vi "Example_scatter.vi"() -> ()   [LabVIEW 8.6]
uses:
  Controls/lxw_chart_marker_type.ctl
  Controls/lxw_chart_legend_position.ctl
  Controls/lxw_chart_axis_type.ctl
  Controls/lxw_chart_type.ctl
panel:
  out "function return 2":string
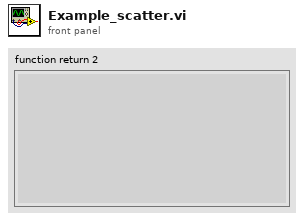
[diagram p1: front panel]
types:
  T1 = enum32{"invalid app kind", "Development System", "Run Time System", "Student Edition", "Embedded LabVIEW", "Evaluation", "Custom"}
  T2 = cluster{"color":u32, "none":u8, "@dummy control@":i8, "@dummy control@":i8, "@dummy control@":i8, "width":sgl, "dash_type":u8, "transparency":u8}
  T3 = cluster{"color":u32, "none":u8, "transparency":u8}
  T4 = typedef "lxw_chart_type.ctl" = u8
  T5 = typedef "lxw_chart_axis_type.ctl" = u8
  T6 = typedef "lxw_chart_legend_position.ctl" = u8
  T7 = typedef "lxw_chart_marker_type.ctl" = u8
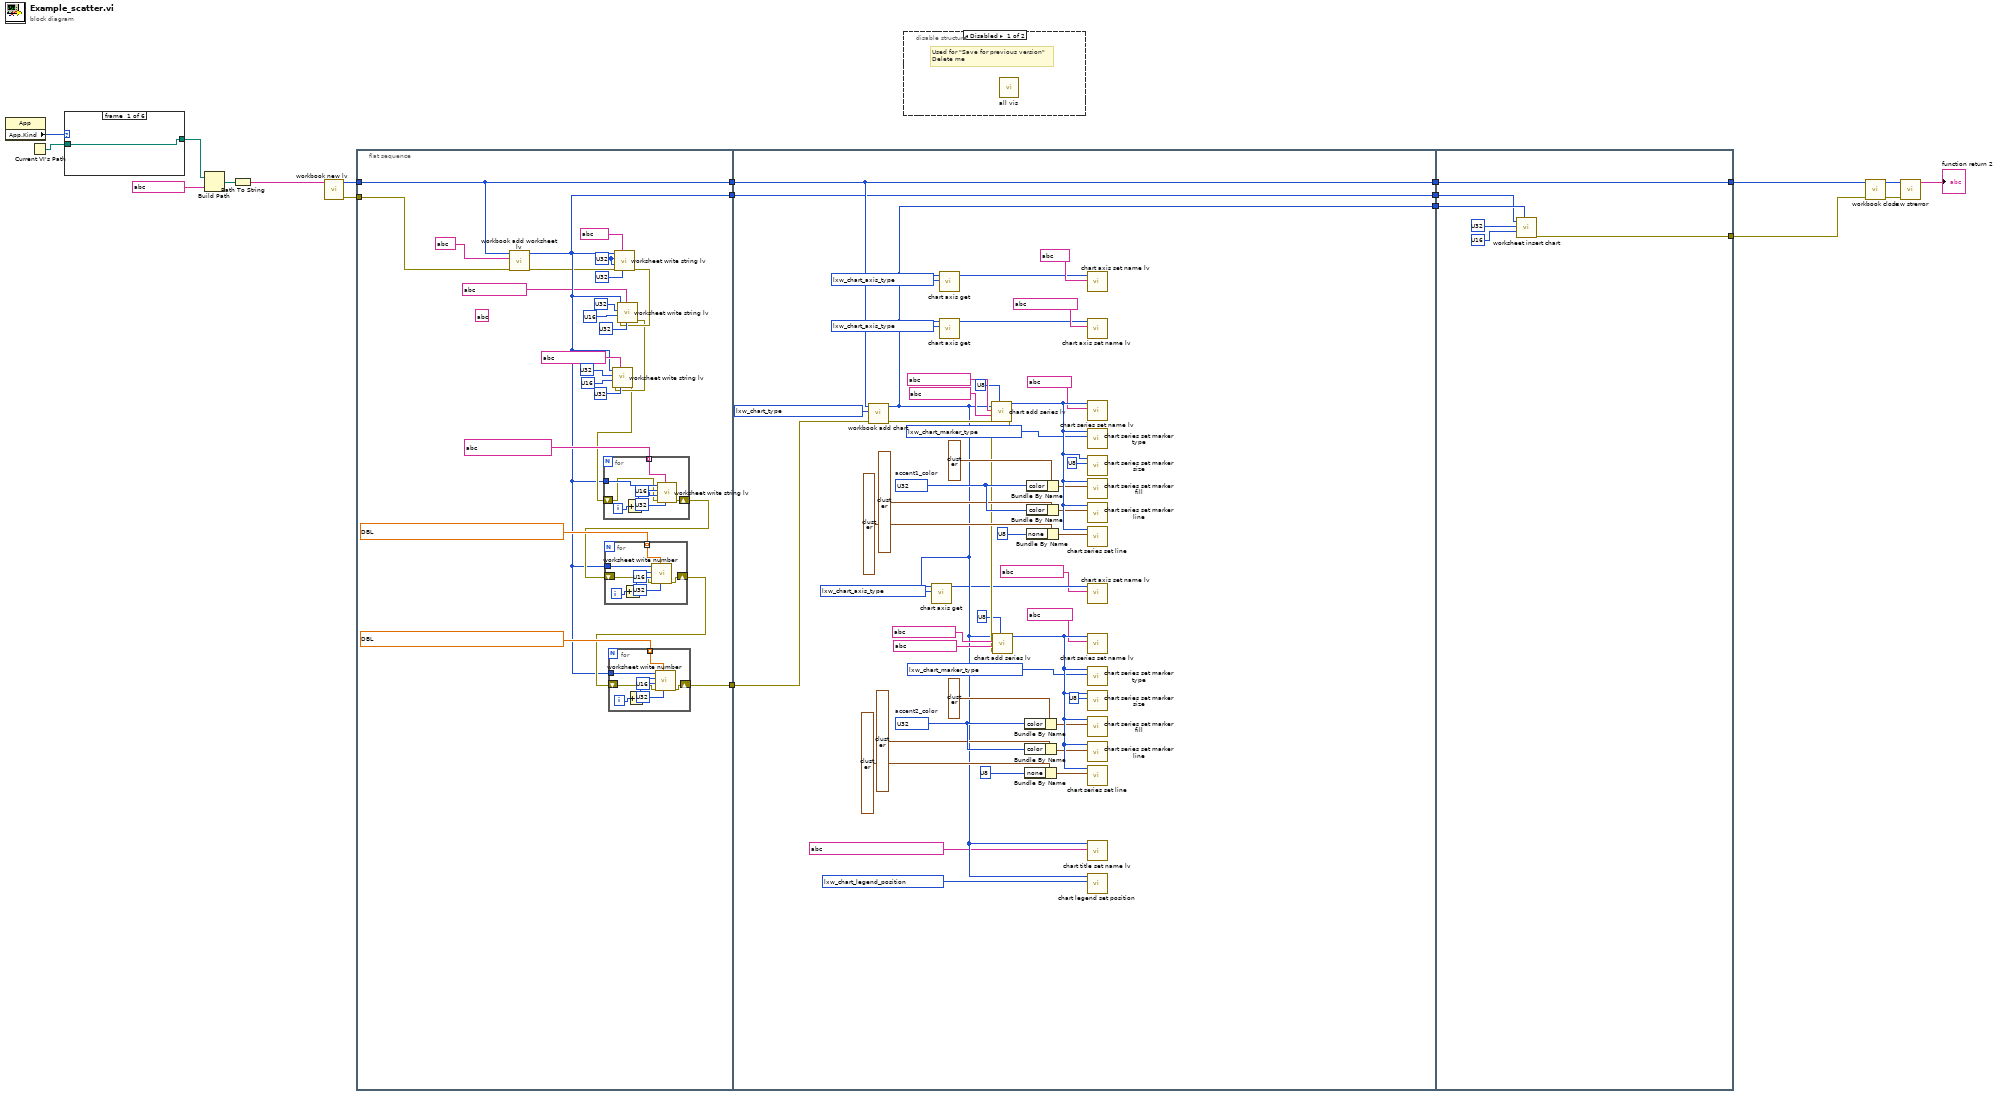
[diagram p0: block diagram]
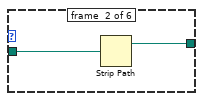
[diagram p2: hidden frame]
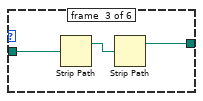
[diagram p3: hidden frame]
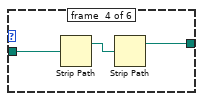
[diagram p4: hidden frame]
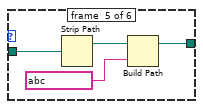
[diagram p5: hidden frame]
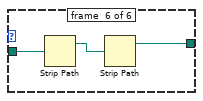
[diagram p6: hidden frame]
diagram:
  n1 = property class="App"() -> ("App.Kind"=w6:T1)  [unwired: 2 in, 2 out]
  n2 = Current VI's Path() -> (path=w5:path)
  n3 = case shown="\"Evaluation\"" w6 {
    tunnel: w5 -> [w20 w22 w25 w28 w32 w35]
    tunnel: [w20 w21 w23 w26 w30 w33] -> w4
    frame #0 {
    }
    frame #1 {
      n4 = Strip Path(path=w22) -> (stripped path=w21:path)  [unwired: 1 out]
    }
    frame #2 {
      n5 = Strip Path(path=w25) -> (stripped path=w24:path)  [unwired: 1 out]
      n6 = Strip Path(path=w24) -> (stripped path=w23:path)  [unwired: 1 out]
    }
    frame #3 {
      n7 = Strip Path(path=w28) -> (stripped path=w27:path)  [unwired: 1 out]
      n8 = Strip Path(path=w27) -> (stripped path=w26:path)  [unwired: 1 out]
    }
    frame #4 {
      n9 = Strip Path(path=w32) -> (stripped path=w31:path)  [unwired: 1 out]
      n10 = Build Path(base path=w31, name or relative path=string ?) -> (appended path=w30:path)
    }
    frame #5 {
      n11 = Strip Path(path=w35) -> (stripped path=w34:path)  [unwired: 1 out]
      n12 = Strip Path(path=w34) -> (stripped path=w33:path)  [unwired: 1 out]
    }
  }
  n13 = Build Path(base path=w4, name or relative path=string ? ("filename")) -> (appended path=w2:path)
  n14 = Path To String(path=w2) -> (string=w1:string)
  n15 = call "workbook new lv.vi"("filename"=w1) -> ("error out"=w17:errorcluster, "function return"=w19:u32)  [unwired: 9 in]
  n16 = flat-sequence {
    tunnel: w19 -> [w40]
    tunnel: w17 -> [w37]
    tunnel: [w41] -> w16
    tunnel: [w40] -> w9
    tunnel: [w39] -> w7
    tunnel: w16 -> [w111]
    tunnel: [w112] -> w14
    tunnel: [w99] -> w13
    tunnel: w9 -> [w112]
    tunnel: [w96] -> w8
    tunnel: w7 -> [w96]
    tunnel: [w136] -> w15
    tunnel: w14 -> [w137]
    tunnel: w13 -> [w138]
    tunnel: [w137] -> w12
    tunnel: w8 -> [w133]
    frame #0 {
      (unwired) string ?
      w59 = u32 ? ("row")
      n17 = call "workbook add worksheet lv.vi"("error in (no error)"=w37, "sheetname"=string ?, "workbook"=w40) -> ("error out"=w36:errorcluster, "function return"=w39:u32)  [unwired: 7 in]
      n18 = call "worksheet write string lv.vi"("format"=u32 ?, "string"=string ?, "error in (no error)"=w36, "col"=w59, "row"=w59, "worksheet"=w39) -> ("error out"=w46:errorcluster)  [unwired: 4 in, 1 out]
      n19 = call "worksheet write string lv.vi"("format"=u32 ?, "string"=string ?, "error in (no error)"=w46, "col"=u16 ?, "row"=u32 ?, "worksheet"=w39) -> ("error out"=w45:errorcluster)  [unwired: 4 in, 1 out]
      n20 = call "worksheet write string lv.vi"("format"=u32 ?, "string"=string ?, "error in (no error)"=w45, "col"=u16 ?, "row"=u32 ?, "worksheet"=w39) -> ("error out"=w44:errorcluster)  [unwired: 4 in, 1 out]
      n21 = for {
        tunnel: w39 -> [w84]
        tunnel: string[] ? -> [w79] mode=indexing
        shift-right: [w77] -> w43
        shift-left: w44 -> [w78]
        i -> [w83]
        n22 = Increment(x=w83) -> (x+1=w82:i32)
        n23 = call "worksheet write string lv.vi"("format"=u32 ?, "string"=w79, "error in (no error)"=w78, "col"=u16 ?, "row"=w82, "worksheet"=w84) -> ("error out"=w77:errorcluster)  [unwired: 4 in, 1 out]
      }
      n24 = for {
        tunnel: w39 -> [w76]
        tunnel: dbl[] ? -> [w75] mode=indexing
        shift-right: [w69] -> w42
        shift-left: w43 -> [w70]
        i -> [w74]
        n25 = Increment(x=w74) -> (x+1=w73:i32)
        n26 = call "worksheet write number.vi"("format"=u32 ?, "number"=w75, "error in (no error)"=w70, "col"=u16 ?, "row"=w73, "worksheet"=w76) -> ("error out"=w69:errorcluster)  [unwired: 4 in, 1 out]
      }
      n27 = for {
        tunnel: w39 -> [w68]
        tunnel: dbl[] ? -> [w67] mode=indexing
        shift-right: [w61] -> w41
        shift-left: w42 -> [w62]
        i -> [w66]
        n28 = Increment(x=w66) -> (x+1=w65:i32)
        n29 = call "worksheet write number.vi"("format"=u32 ?, "number"=w67, "error in (no error)"=w62, "col"=u16 ?, "row"=w65, "worksheet"=w68) -> ("error out"=w61:errorcluster)  [unwired: 4 in, 1 out]
      }
    }
    frame #1 {
      w85 = T4 ? items=["LXW_CHART_NONE", "LXW_CHART_AREA", "LXW_CHART_AREA_STACKED", "LXW_CHART_AREA_STACKED_PERCENT", "LXW_CHART_BAR", "LXW_CHART_BAR_STACKED", "LXW_CHART_BAR_STACKED_PERCENT", "LXW_CHART_COLUMN", "LXW_CHART_COLUMN_STACKED", "LXW_CHART_COLUMN_STACKED_PERCENT", "LXW_CHART_DOUGHNUT", "LXW_CHART_LINE", "LXW_CHART_LINE_STACKED", "LXW_CHART_LINE_STACKED_PERCENT", "LXW_CHART_PIE", "LXW_CHART_SCATTER", "LXW_CHART_SCATTER_STRAIGHT", "LXW_CHART_SCATTER_STRAIGHT_WITH_MARKERS", "LXW_CHART_SCATTER_SMOOTH", "LXW_CHART_SCATTER_SMOOTH_WITH_MARKERS", "LXW_CHART_RADAR", "LXW_CHART_RADAR_WITH_MARKERS", "LXW_CHART_RADAR_FILLED", "LXW_CHART_STOCK"] ("chart_type")
      w90 = T5 ? items=["LXW_CHART_AXIS_TYPE_X", "LXW_CHART_AXIS_TYPE_Y", "LXW_CHART_AXIS_TYPE_X2", "LXW_CHART_AXIS_TYPE_Y2"] ("axis_type")
      w91 = T5 ? items=["LXW_CHART_AXIS_TYPE_X", "LXW_CHART_AXIS_TYPE_Y", "LXW_CHART_AXIS_TYPE_X2", "LXW_CHART_AXIS_TYPE_Y2"] ("axis_type")
      w92 = T5 ? items=["LXW_CHART_AXIS_TYPE_X", "LXW_CHART_AXIS_TYPE_Y", "LXW_CHART_AXIS_TYPE_X2", "LXW_CHART_AXIS_TYPE_Y2"] ("axis_type")
      w97 = T6 ? items=["LXW_CHART_LEGEND_NONE", "LXW_CHART_LEGEND_RIGHT", "LXW_CHART_LEGEND_LEFT", "LXW_CHART_LEGEND_TOP", "LXW_CHART_LEGEND_BOTTOM", "LXW_CHART_LEGEND_TOP_RIGHT", "LXW_CHART_LEGEND_OVERLAY_RIGHT", "LXW_CHART_LEGEND_OVERLAY_LEFT"] ("position")
      w119 = T7 ? items=["LXW_CHART_MARKER_AUTOMATIC", "LXW_CHART_MARKER_NONE", "LXW_CHART_MARKER_SQUARE", "LXW_CHART_MARKER_DIAMOND", "LXW_CHART_MARKER_TRIANGLE", "LXW_CHART_MARKER_X", "LXW_CHART_MARKER_STAR", "LXW_CHART_MARKER_SHORT_DASH", "LXW_CHART_MARKER_LONG_DASH", "LXW_CHART_MARKER_CIRCLE", "LXW_CHART_MARKER_PLUS"] ("type")
      w118 = T7 ? items=["LXW_CHART_MARKER_AUTOMATIC", "LXW_CHART_MARKER_NONE", "LXW_CHART_MARKER_SQUARE", "LXW_CHART_MARKER_DIAMOND", "LXW_CHART_MARKER_TRIANGLE", "LXW_CHART_MARKER_X", "LXW_CHART_MARKER_STAR", "LXW_CHART_MARKER_SHORT_DASH", "LXW_CHART_MARKER_LONG_DASH", "LXW_CHART_MARKER_CIRCLE", "LXW_CHART_MARKER_PLUS"] ("type")
      w129 = u32 ?  # accent2_color
      w123 = u32 ?  # accent1_color
      n30 = call "workbook add chart.vi"("error in (no error)"=w111, "chart_type"=w85, "workbook"=w112) -> ("error out"=w110:errorcluster, "function return"=w99:u32)  [unwired: 7 in]
      n31 = call "chart axis get.vi"("axis_type"=w90, "chart"=w99) -> ("function return"=w94:u32)  [unwired: 8 in, 1 out]
      n32 = call "chart axis get.vi"("axis_type"=w91, "chart"=w99) -> ("function return"=w89:u32)  [unwired: 8 in, 1 out]
      n33 = call "chart axis get.vi"("axis_type"=w92, "chart"=w99) -> ("function return"=w88:u32)  [unwired: 8 in, 1 out]
      n34 = call "chart add series lv.vi"("y2_axis"=u8 ?, "error in (no error)"=w110, "values"=string ?, "categories"=string ?, "chart"=w99) -> ("error out"=w109:errorcluster, "function return"=w132:u32)  [unwired: 5 in]
      n35 = call "chart add series lv.vi"("y2_axis"=u8 ?, "error in (no error)"=w109, "values"=string ?, "categories"=string ?, "chart"=w99) -> ("function return"=w130:u32)  [unwired: 5 in, 1 out]
      n36 = Bundle By Name(cluster=T3 ? ("fill"), "color"=w129) -> (w103:T3)
      n37 = Bundle By Name(cluster=T2 ? ("line"), "color"=w129) -> (w101:T2)
      n38 = Bundle By Name(cluster=T2 ? ("line"), "none"=u8 ?) -> (w102:T2)
      n39 = Bundle By Name(cluster=T3 ? ("fill"), "color"=w123) -> (w107:T3)
      n40 = Bundle By Name(cluster=T2 ? ("line"), "color"=w123) -> (w106:T2)
      n41 = Bundle By Name(cluster=T2 ? ("line"), "none"=u8 ?) -> (w105:T2)
      n42 = call "chart axis set name lv.vi"("name"=string ?, "axis"=w89) -> ()  [unwired: 9 in, 1 out]
      n43 = call "chart axis set name lv.vi"("name"=string ?, "axis"=w88) -> ()  [unwired: 9 in, 1 out]
      n44 = call "chart series set name lv.vi"("name"=string ?, "series"=w132) -> ()  [unwired: 9 in, 1 out]
      n45 = call "chart series set marker type.vi"("type"=w118, "series"=w132) -> ()  [unwired: 9 in, 1 out]
      n46 = call "chart series set marker size.vi"("size"=u8 ?, "series"=w132) -> ()  [unwired: 9 in, 1 out]
      n47 = call "chart series set marker fill.vi"("fill"=w107, "series"=w132) -> ()  [unwired: 8 in, 2 out]
      n48 = call "chart series set marker line.vi"("line"=w106, "series"=w132) -> ()  [unwired: 8 in, 2 out]
      n49 = call "chart series set line.vi"("line"=w105, "series"=w132) -> ()  [unwired: 8 in, 2 out]
      n50 = call "chart axis set name lv.vi"("name"=string ?, "axis"=w94) -> ()  [unwired: 9 in, 1 out]
      n51 = call "chart series set name lv.vi"("name"=string ?, "series"=w130) -> ()  [unwired: 9 in, 1 out]
      n52 = call "chart series set marker type.vi"("type"=w119, "series"=w130) -> ()  [unwired: 9 in, 1 out]
      n53 = call "chart series set marker size.vi"("size"=u8 ?, "series"=w130) -> ()  [unwired: 9 in, 1 out]
      n54 = call "chart series set marker fill.vi"("fill"=w103, "series"=w130) -> ()  [unwired: 8 in, 2 out]
      n55 = call "chart series set marker line.vi"("line"=w101, "series"=w130) -> ()  [unwired: 8 in, 2 out]
      n56 = call "chart series set line.vi"("line"=w102, "series"=w130) -> ()  [unwired: 8 in, 2 out]
      n57 = call "chart title set name lv.vi"("name"=string ?, "chart"=w99) -> ()  [unwired: 9 in, 1 out]
      n58 = call "chart legend set position.vi"("position"=w97, "chart"=w99) -> ()  [unwired: 9 in, 1 out]
    }
    frame #2 {
      n59 = call "worksheet insert chart.vi"("chart"=w138, "col"=u16 ?, "row"=u32 ?, "worksheet"=w133) -> ("error out"=w136:errorcluster)  [unwired: 6 in, 1 out]
    }
  }
  n60 = disable-structure shown="Disabled" {
    frame #0 {
      # "Used for \"Save for previous version\"\nDelete me"
      n61 = call "all vis.vi"() -> ()  [unwired: 12 in]
    }
    frame #1 {
    }
  }
  n62 = call "workbook close.vi"("error in (no error)"=w15, "workbook"=w12) -> ("error out"=w11:errorcluster, "function return"=w18:u32)  [unwired: 8 in]
  n63 = call "lxw strerror.vi"("error in (no error)"=w11, "error_num"=w18) -> ("function return"=→"function return 2":string)  [unwired: 8 in, 1 out]
